vi "Mindsensors IMU-ACG Config.vi"(10 "Node Data":T1, 11 "NXT":T2) -> ()   [LabVIEW 2010]
uses:
  <vilib>/NXT/Subs/LVHSConnector.ctl
  Datatypes/Node.ctl
  UI Controls/PlugInControls/Pluginbackground.ctl
  <vilib>/Utility/miscctls.llb/LVPointTypeDef.ctl
  <vilib>/NXT/Block Support/HWPage.SensorMode.ctl
  <vilib>/NXT/Block Support/HWPage.SensorType.ctl
  ConvertNodeAddrSensor.vi
panel:
  out "Heading":i16
  in  "Heading":string
  in  "Mag":string
  out "Z:":i16
  out "Y:":i16
  out "X:":i16
  in  "Gyro":string
  out "Z:":i16
  out "Y:":i16
  out "X:":i16
  out "Z:":i16
  out "Y:":i16
  out "X:":i16
  in  "Accel":string
  in  "Tilt":string
  out "Z:":i8
  in  "Sensor Readings:":string
  out "Y:":i8
  out "X:":i8
  in  "Device Addr":u8 format="%x"
  out "?":dbl format="%#.2g"
  out "number":i8
  in  "Device Address":string
  in  "NXT Port":string
  in  "Name":string
  out "Headline":string="Type (auto populated)"
  in  "Sensor Parameters":string
  in  "Instance Specific Data":cluster{"Example Data":dbl}
  in  "Reset":bool
  in  "Save":bool
  in  "Stop":bool
  out "Background":T3=TRUE
  # "<- No controls below this line"
  # "Common controls such as Buttons, Rings, Sliders, Graphs, Decorations, etc can be found in the <labview>\\Targets\\NI\\NXT\\NXT Toolkit\\Schematic Editor\\UI Controls\\Plugin Controls\\ folder. Use these controls when possible to ensure a consistent look and feel with LabVIEW Education Edition."
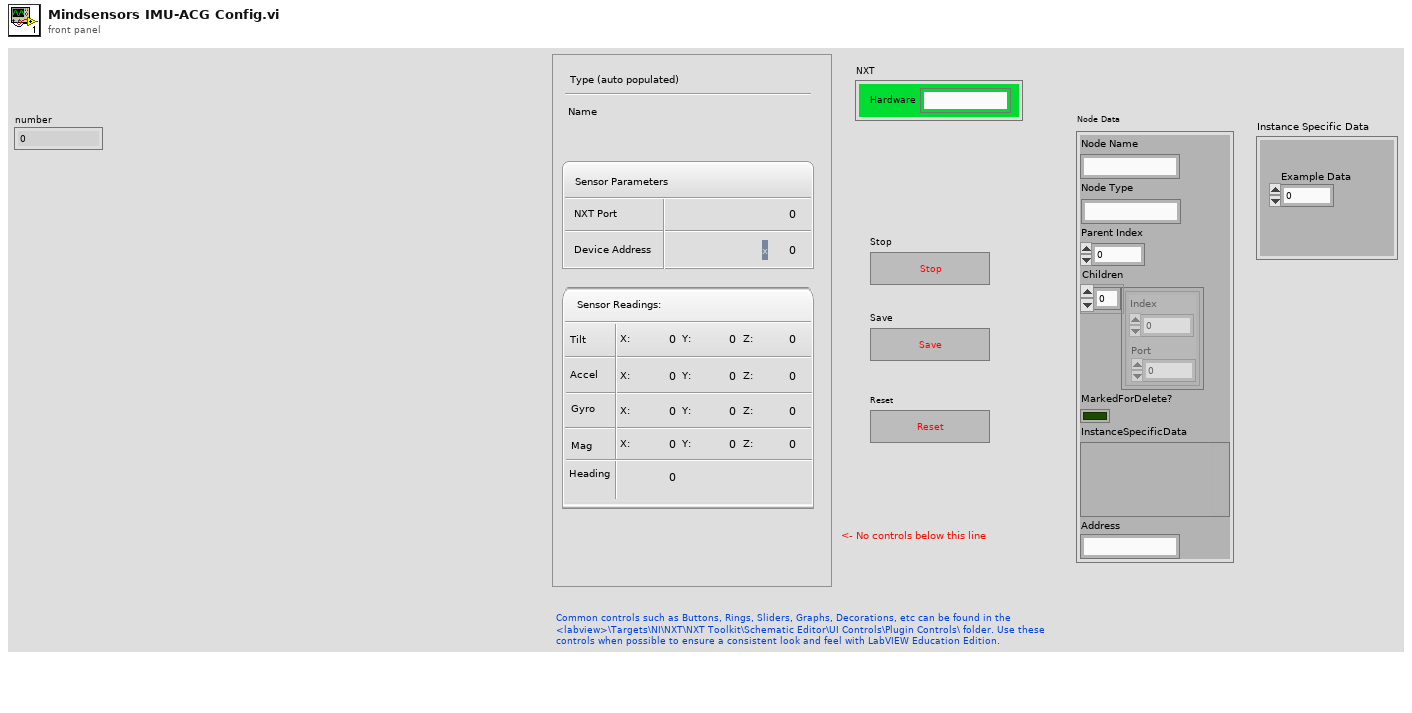
[diagram p1: front panel]
types:
  T1 = typedef "Node.ctl" = cluster{"Node Name":string, "Node Type":string, "Parent Index":i16, "Children":cluster{"Index":u16, "Port":u16}[], "MarkedForDelete?":bool, "InstanceSpecificData":variant, "Address":string}
  T2 = typedef "LVHSConnector.ctl" = cluster{"Hardware":string, "Flattened String":string}
  T3 = typedef "Pluginbackground.ctl" = bool
  T4 = typedef "LVPointTypeDef.ctl" = cluster{"Horizontal":i16, "Vertical":i16}
  T5 = enum8{"Enabled", "Disabled", "Disabled and Grayed Out"}
  T6 = typedef "HWPage.SensorMode.ctl" = u8
  T7 = typedef "HWPage.SensorType.ctl" = u8
  T8 = typedef "NXT_InputPort.ctl" = u8
  T9 = typedef "nxt.ctl" = cluster{"nxtHandle":u32, "fileHandle":u32, "fileIterHandle":u32, "moduleHandle":u32, "modIterHandle":u32, "nxtIterHandle":u32}
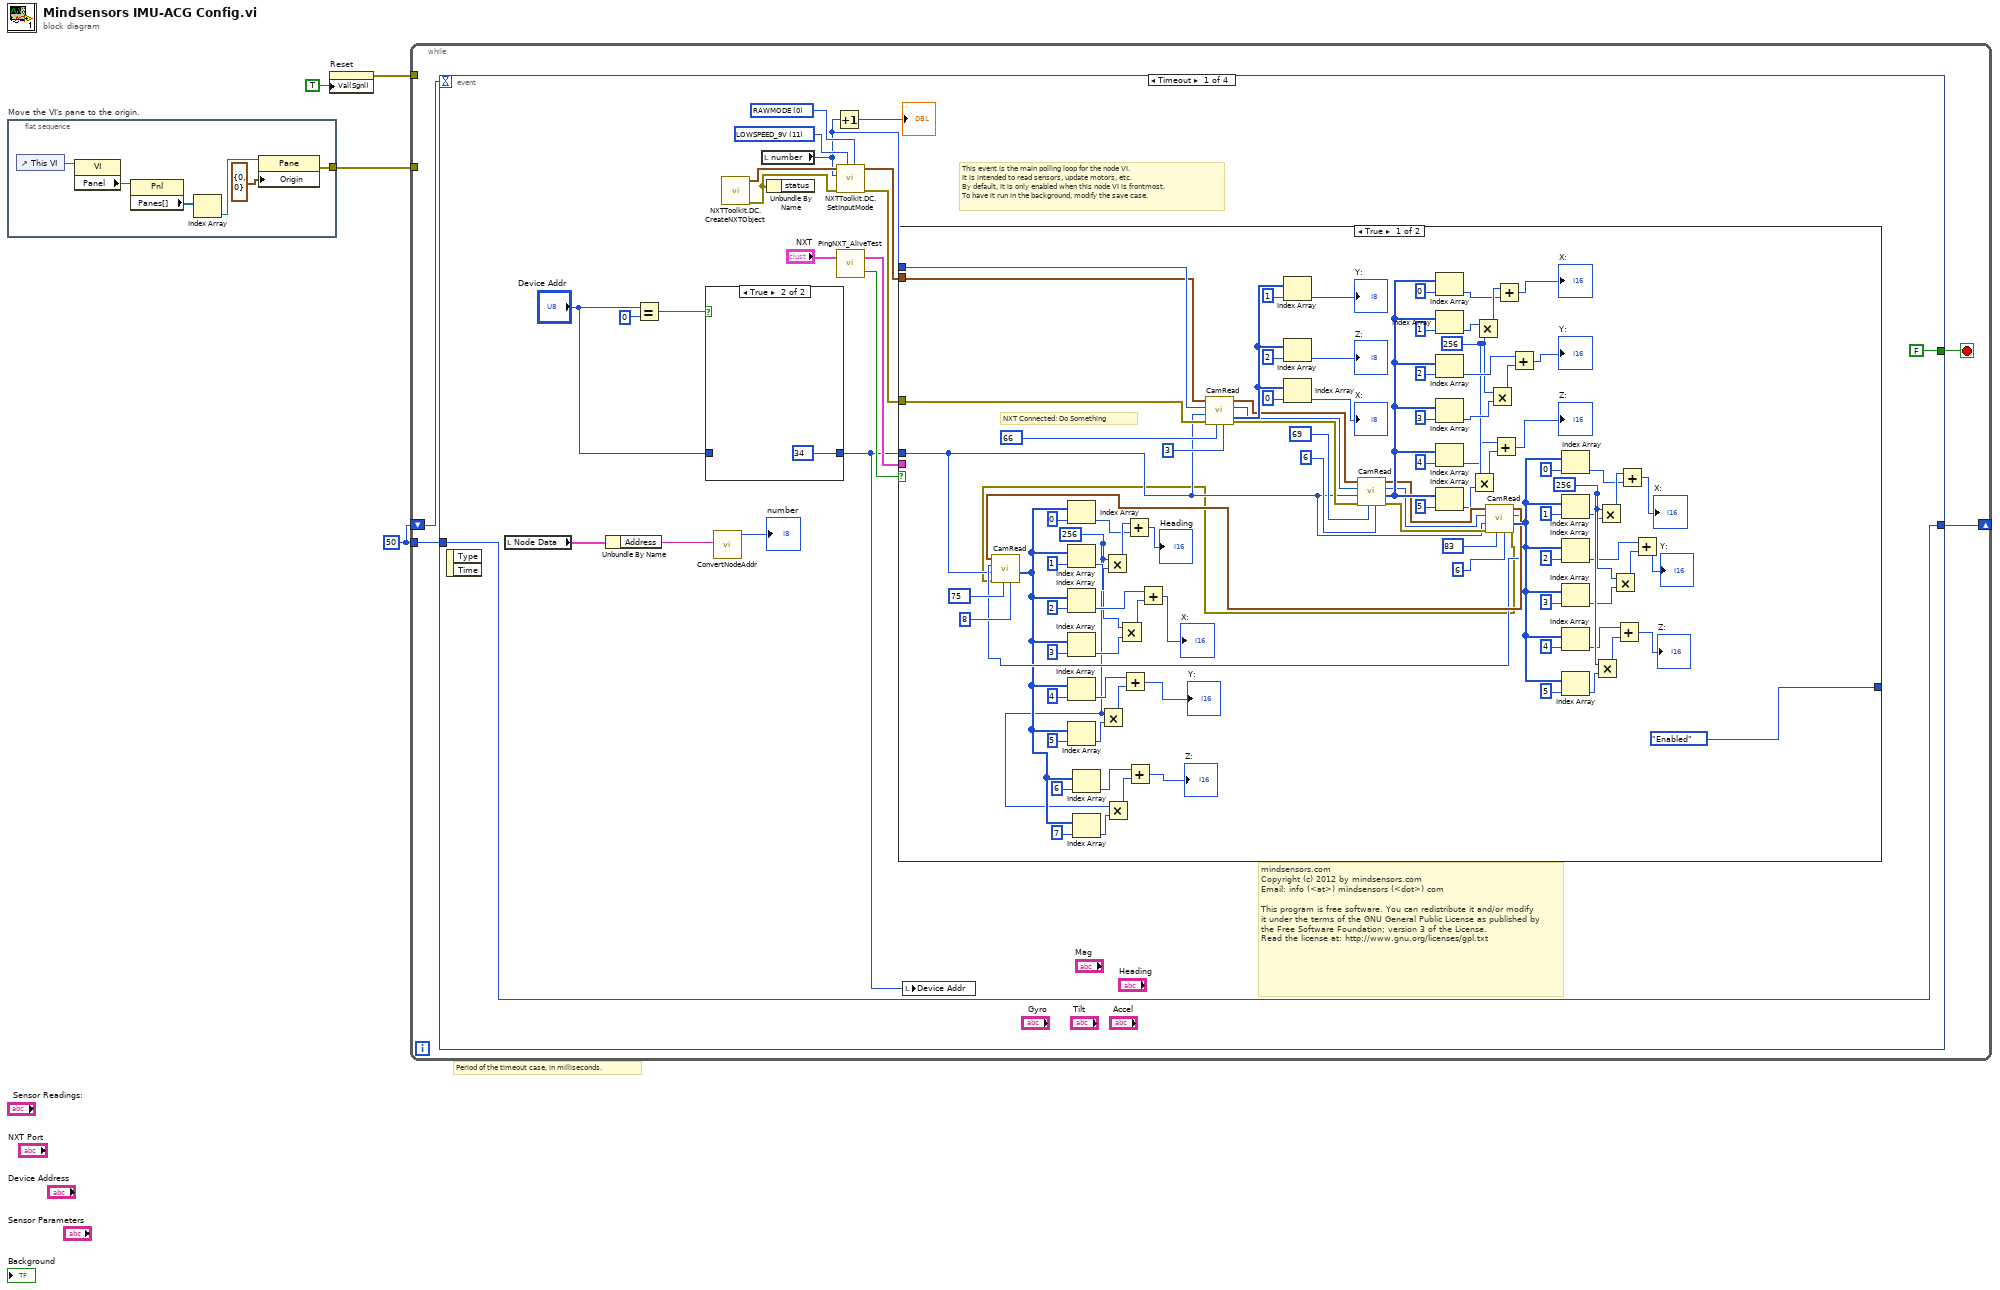
[diagram p0: block diagram]
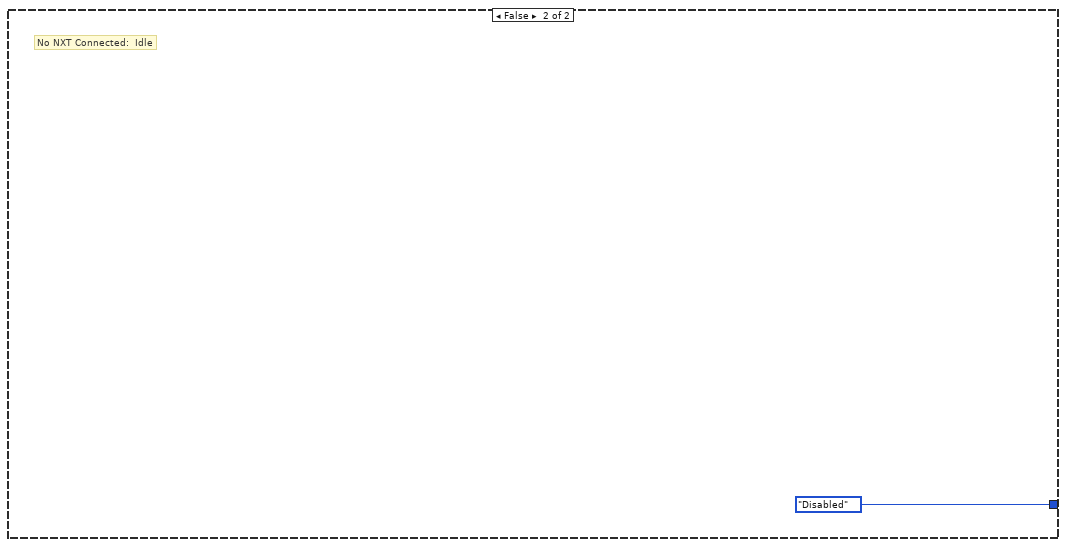
[diagram p3: hidden frame]
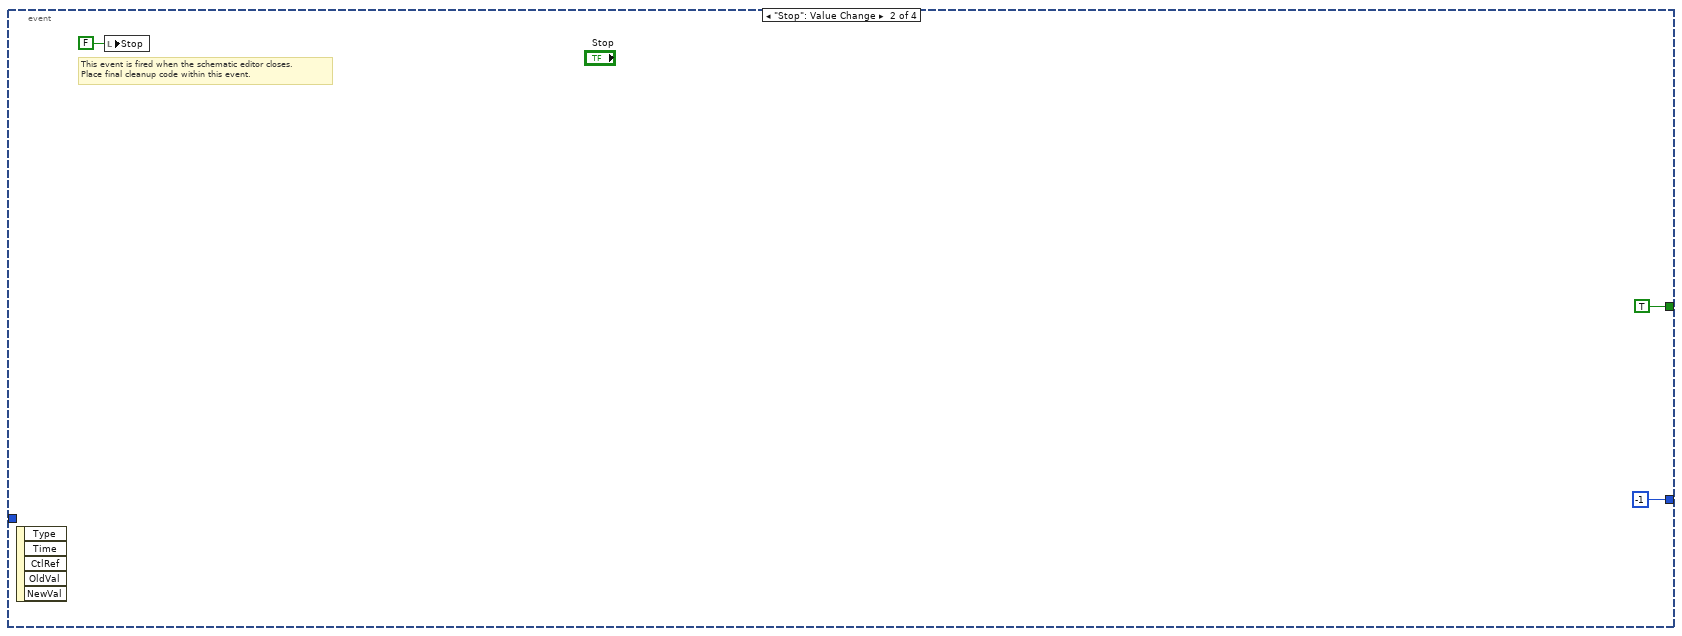
[diagram p4: hidden frame]
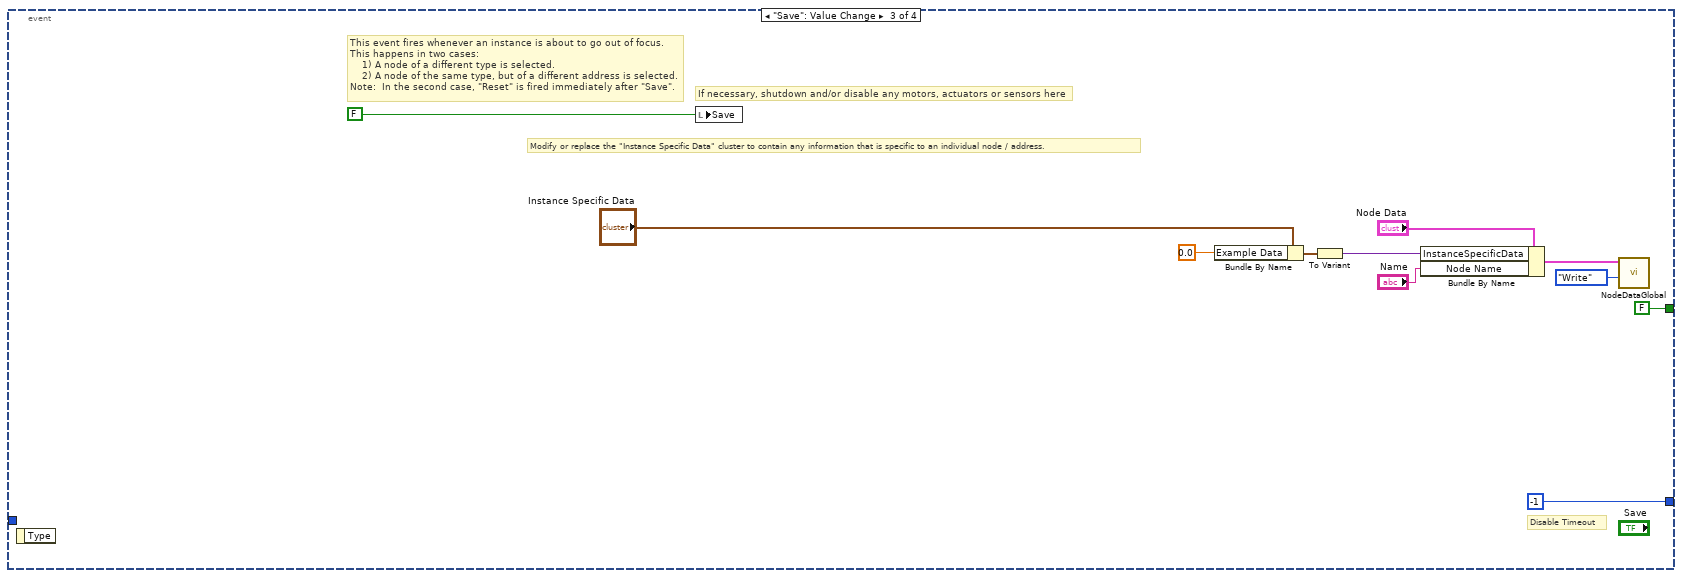
[diagram p5: hidden frame]
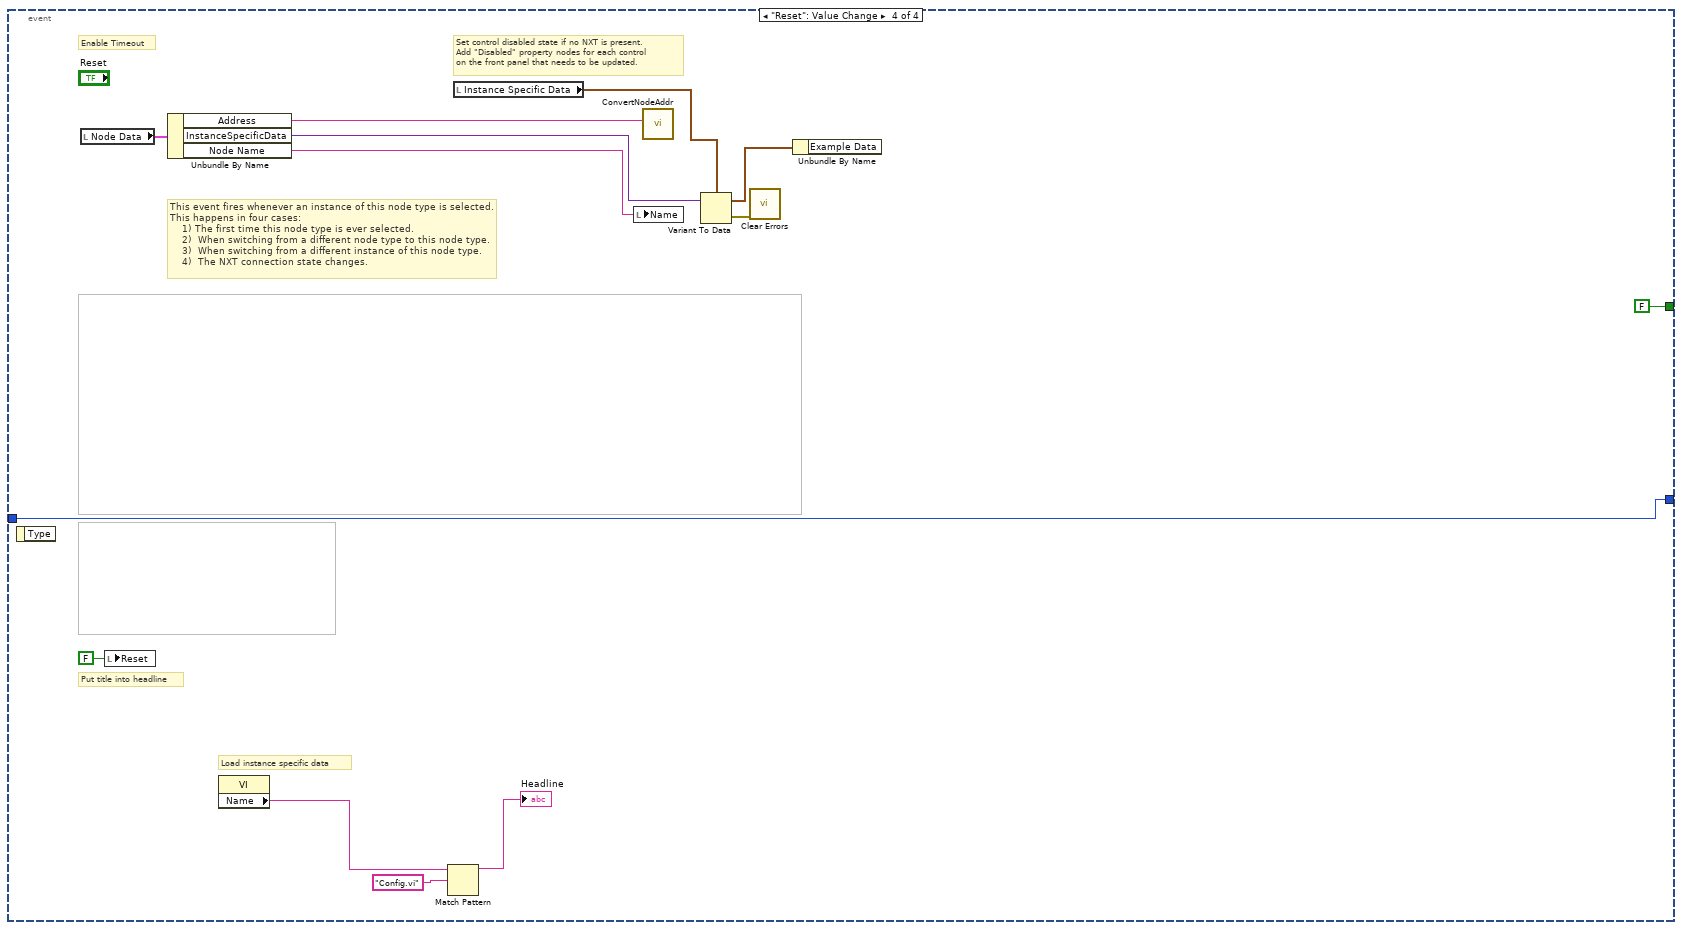
[diagram p6: hidden frame]
diagram:
  w2 = 50
  # "Period of the timeout case, in milliseconds."
  n1 = flat-sequence "Move the VI's pane to the origin." {
    tunnel: [w5] -> w1
    frame #0 {
      n2 = control-ref of="This VI"() -> (w6:refnum<vi>)
      n3 = property class="VI"(reference=w6) -> ("Panel"=w7:refnum<vi>)  [unwired: 1 in, 2 out]
      n4 = property class="Pnl"(reference=w7) -> ("Panes[]"=w8:refnum<vi>[])  [unwired: 1 in, 2 out]
      n5 = Index Array(array=w8) -> (element=w9:refnum<vi>)  [unwired: 1 in]
      n6 = property class="Pane"(reference=w9, "Origin"=T4 {"Horizontal"=0, "Vertical"=0}) -> (error out=w5:errorcluster)  [unwired: 1 in, 1 out]
    }
  }
  n7 = property on="Reset" class="Bool (strict)"("Val(Sgnl)"=TRUE ("Value (Signaling)")) -> (error out=w3:errorcluster)  [unwired: 2 in, 1 out]
  n8 = while {
    tunnel: w3 -> [_]
    shift-right: [w12] -> _
    shift-left: w2 -> [w13]
    tunnel: w2 -> [w11]
    tunnel: w1 -> [_]
    stop <- w14 stop-if-true
    n9 = event shown="[0] Timeout" {
      selector: _ -> [_ _ _ _]
      dyn-events: _ -> [_ _ _ _]
      timeout: w13 -> [_ _ _ _]
      tunnel: [FALSE TRUE FALSE FALSE] -> w14
      tunnel: [w33 -1 -1 w155] -> w12
      tunnel: w11 -> [w33 _ _ w155]
      event Timeout {
        w28 = T6 0 items=["RAWMODE"=0, "BOOLEANMODE"=32, "TRANSITIONCNTMODE"=64, "PERIODCOUNTERMODE"=96, "PCTFULLSCALEMODE"=128, "CELSIUSMODE"=160, "FAHRENHEITMODE"=192, "ANGLESTEPMODE"=224] ("Sensor Mode (RAWMODE)")
        w27 = T7 11 items=["NO_SENSOR", "SWITCH", "TEMPERATURE", "REFLECTION", "ANGLE", "LIGHT_ACTIVE", "LIGHT_INACTIVE", "SOUND_DB", "SOUND_DBA", "CUSTOM", "LOWSPEED", "LOWSPEED_9V", "HIGHSPEED"] ("Sensor Type (NO_SENSOR)")
        # "mindsensors.com\nCopyright (c) 2012 by mindsensors.com\nEmail: info (<at>) mindsensors (<dot>) com\n\nThis program is free software. You can redistribute it and/or modify\nit under the terms of the GNU General Public License as published by\nthe Free Software Foundation; version 3 of the License.\nRead the license at: http://www.gnu.org/licenses/gpl.txt"
        # "This event is the main polling loop for the node VI.\nIt is intended to read sensors, update motors, etc.\nBy default, it is only enabled when this node VI is frontmost.\nTo have it run in the background, modify the save case."
        n10 = event-data() -> ()  [unwired: 1 in, 2 out]
        n11 = local read "Node Data"() -> (w31:T1)
        n12 = Unbundle By Name(w31) -> ("Address"=w18:string)
        n13 = Equal?(x="Device Addr", y=u8 0) -> (x = y?=w21:bool)
        n14 = case shown="True" w21 {
          tunnel: [w35 u8 34 ("Device Addr 2")] -> w20
          tunnel: "Device Addr" -> [w35 _]
          frame False {
          }
          frame True {
          }
        }
        n15 = call-poly "ConvertNodeAddr.vi"("Sensor Port"=w18) -> ("NXT Port"=→"number":T8)  [unwired: 6 in, 4 out]
        n16 = call <vilib>:"NXTToolkit.DC.CreateNXTObject.vi"() -> ("error out"=w25:errorcluster, "NXTObject"=w26:T9)  [unwired: 9 in, 1 out]
        n17 = local read "number"() -> (w16:i8)
        n18 = Unbundle By Name(w25) -> ()  [unwired: 1 out]
        n19 = Increment(x=w16) -> (x+1=→"?":i8)
        n20 = call <vilib>:"NXTToolkit.DC.SetInputMode.vi"("Sensor Mode (RAWMODE)"=w28, "Sensor Type (NO_SENSOR)"=w27, "error in (no error)"=w25, "Input Port (Port 1)"=w16, "NXTObject"=w26) -> ("error out"=w23:errorcluster, "NXTObject dup"=w24:T9)  [unwired: 4 in, 1 out]
        n21 = call <vilib>:"PingNXT_AliveTest.vi"("NXT"="NXT") -> ("connected?"=w30:bool, "NXT"=w29:T2)  [unwired: 1 in]
        n22 = case shown="True" w30 {
          tunnel: [T5."Enabled" ("Disabled") T5."Disabled" ("Disabled")] -> _
          tunnel: w29 -> [_ _]
          tunnel: w24 -> [w125 _]
          tunnel: w23 -> [w124 _]
          tunnel: w16 -> [w126 _]
          tunnel: w20 -> [w49 _]
          frame True {
            w37 = 256
            w78 = 256
            w85 = 256
            # "NXT Connected: Do Something"
            n23 = call <vilib>:"CamRead.vi"("bytes to read"=u8 3, "Reg Address"=u8 66, "error in (no error)"=w124, "Device Address"=w49, "Input Port in"=w126, "NXTObject"=w125) -> ("error out"=w95:errorcluster, "data Buffer"=w120:u8[], "Input Port out"=w96:T8, "NXTObject dup"=w97:T9)  [unwired: 2 out]
            n24 = Index Array(array=w120, index=1) -> (element=→"Y:":u8)
            n25 = Index Array(array=w120, index=2) -> (element=→"Z:":u8)
            n26 = Index Array(array=w120, index=0) -> (element=→"X:":u8)
            n27 = call <vilib>:"CamRead.vi"("bytes to read"=u8 6, "Reg Address"=u8 69, "error in (no error)"=w95, "Device Address"=w49, "Input Port in"=w96, "NXTObject"=w97) -> ("error out"=w100:errorcluster, "data Buffer"=w110:u8[], "Input Port out"=w99:T8, "NXTObject dup"=w101:T9)  [unwired: 2 out]
            n28 = Index Array(array=w110, index=0) -> (element=w92:u8)
            n29 = Index Array(array=w110, index=1) -> (element=w93:u8)
            n30 = Index Array(array=w110, index=2) -> (element=w88:u8)
            n31 = Index Array(array=w110, index=3) -> (element=w89:u8)
            n32 = Index Array(array=w110, index=4) -> (element=w83:u8)
            n33 = Index Array(array=w110, index=5) -> (element=w84:u8)
            n34 = Multiply(x=w85, y=w84) -> (x*y=w86:i32)
            n35 = Multiply(x=w93, y=w85) -> (x*y=w94:i32)
            n36 = call <vilib>:"CamRead.vi"("bytes to read"=u8 6, "Reg Address"=u8 83, "error in (no error)"=w100, "Device Address"=w49, "Input Port in"=w99, "NXTObject"=w101) -> ("error out"=w48:errorcluster, "data Buffer"=w104:u8[], "Input Port out"=w50:T8, "NXTObject dup"=w51:T9)  [unwired: 2 out]
            n37 = call <vilib>:"CamRead.vi"("bytes to read"=u8 8, "Reg Address"=u8 75, "error in (no error)"=w48, "Device Address"=w49, "Input Port in"=w50, "NXTObject"=w51) -> ("data Buffer"=w42:u8[])  [unwired: 5 out]
            n38 = Index Array(array=w42, index=0) -> (element=w56:u8)
            n39 = Index Array(array=w42, index=1) -> (element=w57:u8)
            n40 = Index Array(array=w42, index=2) -> (element=w55:u8)
            n41 = Index Array(array=w42, index=3) -> (element=w58:u8)
            n42 = Index Array(array=w42, index=4) -> (element=w54:u8)
            n43 = Index Array(array=w42, index=5) -> (element=w59:u8)
            n44 = Index Array(array=w42, index=6) -> (element=w43:u8)
            n45 = Index Array(array=w42, index=7) -> (element=w44:u8)
            n46 = Multiply(x=w37, y=w59) -> (x*y=w60:i32)
            n47 = Multiply(x=w37, y=w57) -> (x*y=w62:i32)
            n48 = Multiply(x=w37, y=w44) -> (x*y=w45:i32)
            n49 = Multiply(x=w37, y=w58) -> (x*y=w61:i32)
            n50 = Add(x=w54, y=w60) -> (x+y=→"Y:":i32)
            n51 = Add(x=w62, y=w56) -> (x+y=→"Heading":i32)
            n52 = Add(x=w43, y=w45) -> (x+y=→"Z:":i32)
            n53 = Add(x=w55, y=w61) -> (x+y=→"X:":i32)
            n54 = Multiply(x=w85, y=w89) -> (x*y=w90:i32)
            n55 = Add(x=w83, y=w86) -> (x+y=→"Z:":i32)
            n56 = Add(x=w94, y=w92) -> (x+y=→"X:":i32)
            n57 = Add(x=w88, y=w90) -> (x+y=→"Y:":i32)
            n58 = Index Array(array=w104, index=0) -> (element=w74:u8)
            n59 = Index Array(array=w104, index=1) -> (element=w75:u8)
            n60 = Index Array(array=w104, index=2) -> (element=w72:u8)
            n61 = Index Array(array=w104, index=3) -> (element=w76:u8)
            n62 = Index Array(array=w104, index=4) -> (element=w70:u8)
            n63 = Index Array(array=w104, index=5) -> (element=w77:u8)
            n64 = Multiply(x=w78, y=w77) -> (x*y=w79:i32)
            n65 = Multiply(x=w78, y=w75) -> (x*y=w81:i32)
            n66 = Multiply(x=w78, y=w76) -> (x*y=w80:i32)
            n67 = Add(x=w70, y=w79) -> (x+y=→"Z:":i32)
            n68 = Add(x=w81, y=w74) -> (x+y=→"X:":i32)
            n69 = Add(x=w72, y=w80) -> (x+y=→"Y:":i32)
          }
          frame False {
            # "No NXT Connected:  Idle"
          }
        }
        n70 = local write "Device Addr"(w20) -> ()
      }
      event "Stop": Value Change {
        # "This event is fired when the schematic editor closes.\nPlace final cleanup code within this event."
        n71 = event-data() -> ()  [unwired: 1 in, 5 out]
        n72 = local write "Stop"(FALSE ("stop")) -> ()
      }
      event "Save": Value Change {
        # "If necessary, shutdown and/or disable any motors, actuators or sensors here"
        # "Modify or replace the \"Instance Specific Data\" cluster to contain any information that is specific to an individual node / address."
        # "Disable Timeout"
        # "This event fires whenever an instance is about to go out of focus.\nThis happens in two cases:\n    1) A node of a different type is selected.\n    2) A node of the same type, but of a different address is selected.\nNote:  In the second case, \"Reset\" is fired immediately after \"Save\"."
        n73 = event-data() -> ()  [unwired: 1 in, 1 out]
        n74 = local write "Save"(FALSE ("stop")) -> ()
        n75 = Bundle By Name(cluster="Instance Specific Data", "Example Data"=0.0) -> (w137:cluster{"Example Data":dbl})
        n76 = To Variant(anything=w137) -> (Variant=w144:variant)
        n77 = Bundle By Name(cluster="Node Data", "InstanceSpecificData"=w144, "Node Name"="Name") -> (w143:T1)
        n78 = call "NodeDataGlobal.vi"("Action"=enum16{"Read", "Write"}."Write", "Node Data In"=w143) -> ()  [unwired: 8 in, 2 out]
      }
      event "Reset": Value Change {
        # "Set control disabled state if no NXT is present.\nAdd \"Disabled\" property nodes for each control\non the front panel that needs to be updated."
        # "Load instance specific data"
        # "Enable Timeout"
        # "This event fires whenever an instance of this node type is selected.\nThis happens in four cases:\n    1) The first time this node type is ever selected.\n    2)  When switching from a different node type to this node type.\n    3)  When switching from a different instance of this node type. \n    4)  The NXT connection state changes."
        # "Put title into headline"
        n79 = event-data() -> ()  [unwired: 1 in, 1 out]
        n80 = local read "Node Data"() -> (w156:T1)
        n81 = local write "Reset"(FALSE ("Reset")) -> ()
        n82 = Unbundle By Name(w156) -> ("Address"=w147:string, "InstanceSpecificData"=w157:variant, "Node Name"=w149:string)
        n83 = property class="VI"() -> ("Name"=w151:string)  [unwired: 2 in, 2 out]
        n84 = Match Pattern(string=w151, regular expression="Config.vi") -> (before substring=→"Headline":string)  [unwired: 1 in, 3 out]
        n85 = local read "Instance Specific Data"() -> (w154:cluster{"Example Data":dbl})
        n86 = local write "Name"(w149) -> ()
        n87 = call-poly "ConvertNodeAddr.vi"("Sensor Port"=w147) -> ()  [unwired: 6 in, 5 out]
        n88 = Variant To Data(Variant=w157, type=w154) -> (error out=w153:errorcluster, data=w148:cluster{"Example Data":dbl})  [unwired: 1 in]
        n89 = call <vilib>:"Clear Errors.vi"("error in (no error)"=w153) -> ()  [unwired: 6 in, 1 out]
        n90 = Unbundle By Name(w148) -> ()  [unwired: 1 out]
      }
    }
  }
